vi "LVJSON Load.vi"(8 "error in (no error)":errorcluster, 11 "JSON in":string) -> (0 "error out":errorcluster, 1 "Empty?":bool, 3 "Root Element out":T1)   [LabVIEW 2019, in "labview_json.lvlib"]
uses:
  labview_json.lvlib
  Element.ctl
  Element Type.ctl
  <vilib>/Utility/error.llb/Error Cluster From Error Code.vi
  <vilib>/ErrorRing/Error Ring.xnode
  <vilib>/regexp/Match Regular Expression.xnode
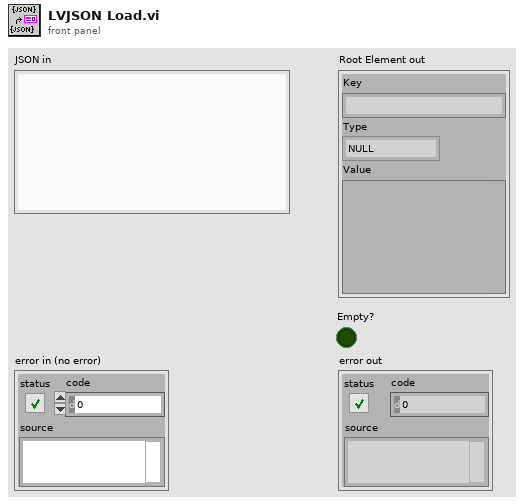
[diagram p1: front panel]
types:
  T1 = typedef "labview_json.lvlib/Element.ctl" = cluster{"Key":string, "Type":T2, "Value":variant}
  T2 = typedef "labview_json.lvlib/Element Type.ctl" = enum8{"NULL", "BOOL", "INT", "UINT", "FLOAT", "STRING", "ARRAY", "OBJECT", "SKIP"}
  T3 = cluster{"Kind":enum8{"Root", "Object", "Array"}, "Name":string, "Values":T1[]}[]
  T4 = cluster{"Kind":enum8{"Root", "Object", "Array"}, "Name":string, "Values":T1[]}
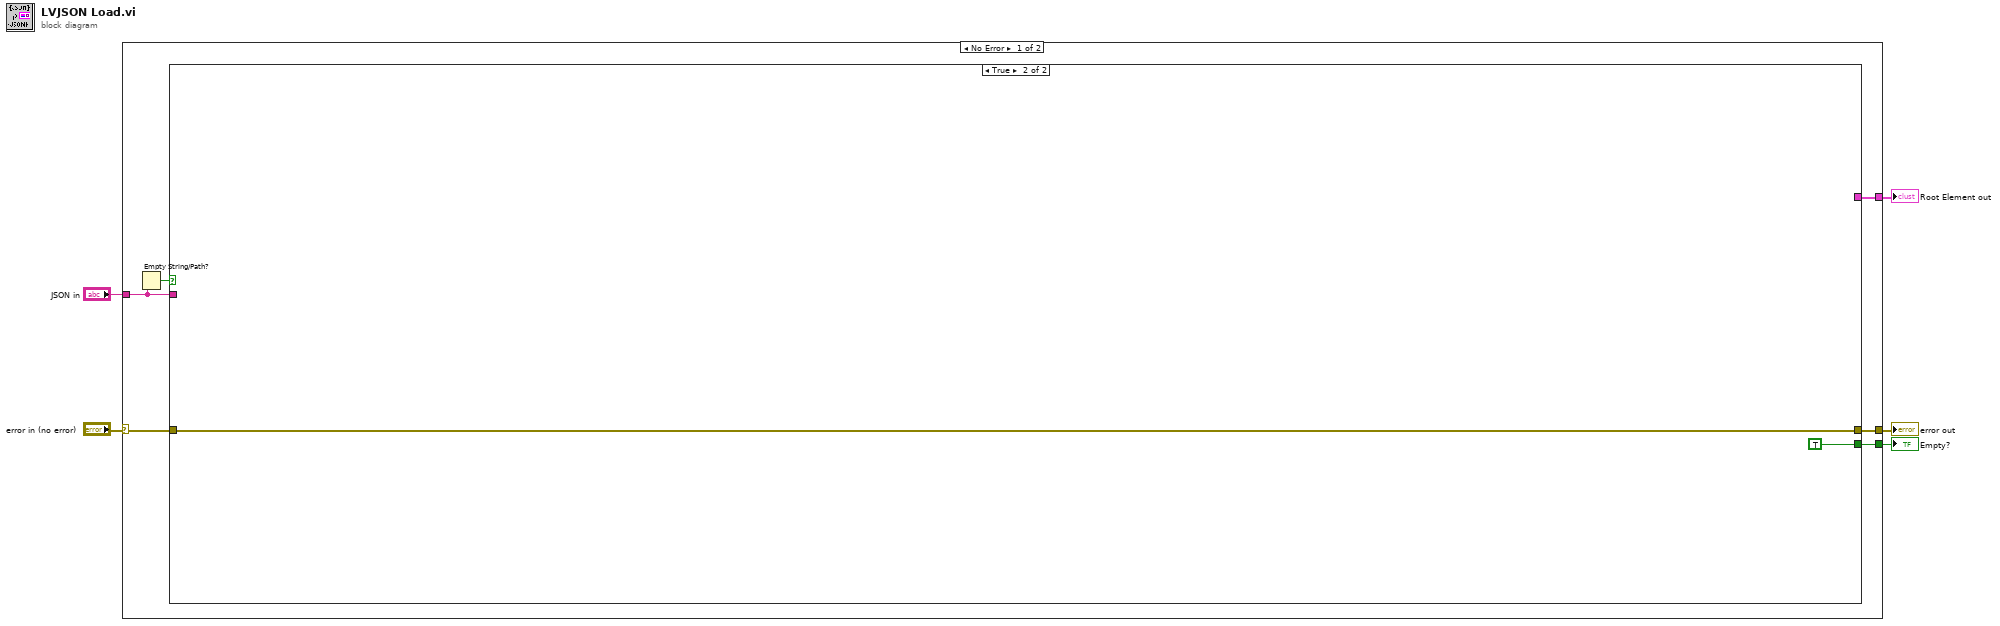
[diagram p0: block diagram]
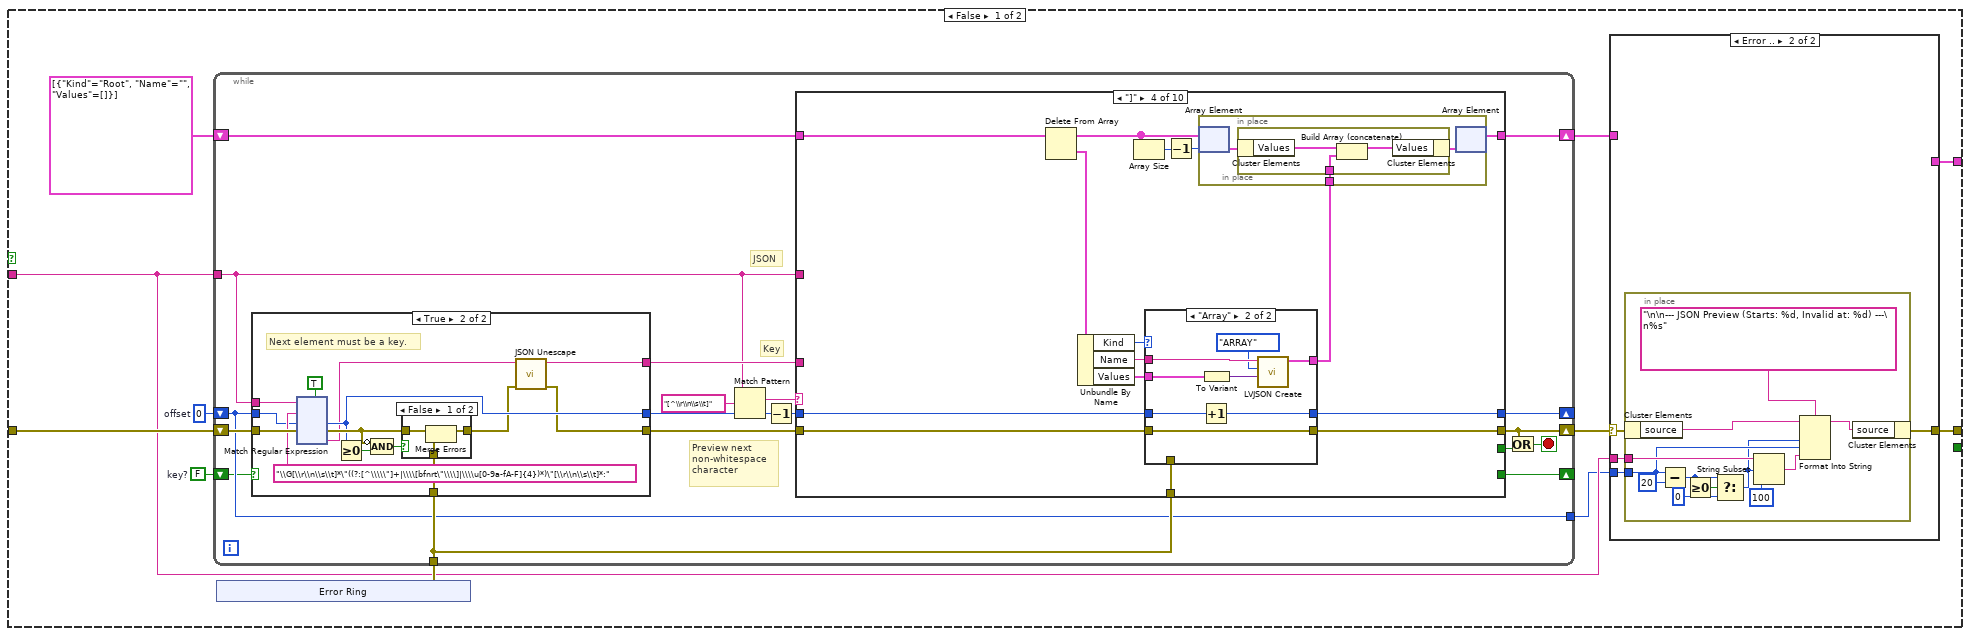
[diagram p2: hidden frame]
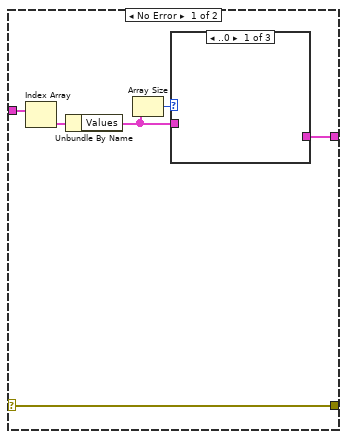
[diagram p3: hidden frame]
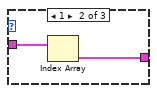
[diagram p4: hidden frame]
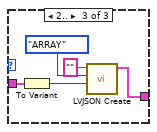
[diagram p5: hidden frame]
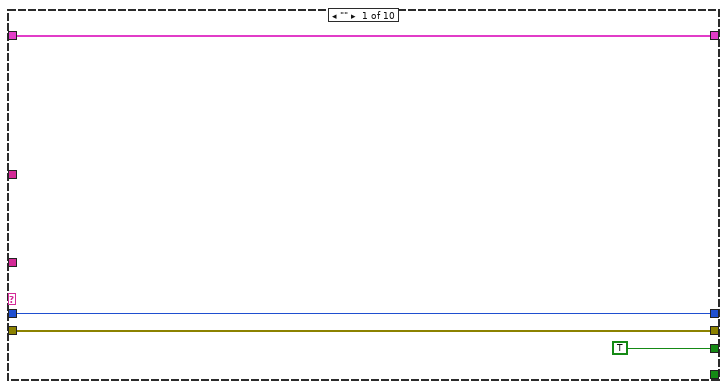
[diagram p8: hidden frame]
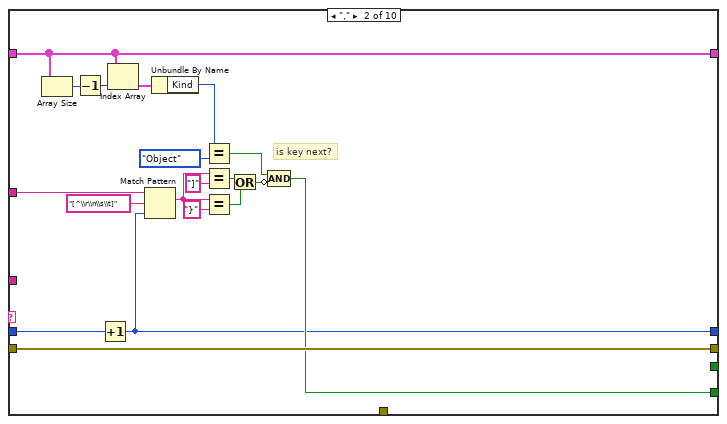
[diagram p9: hidden frame]
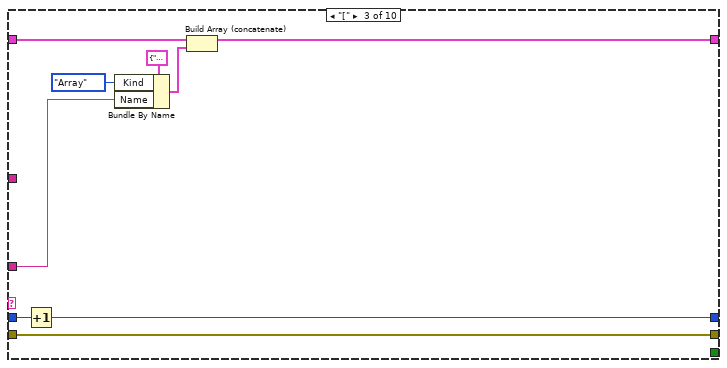
[diagram p10: hidden frame]
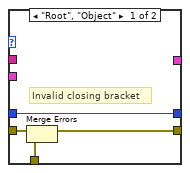
[diagram p11: hidden frame]
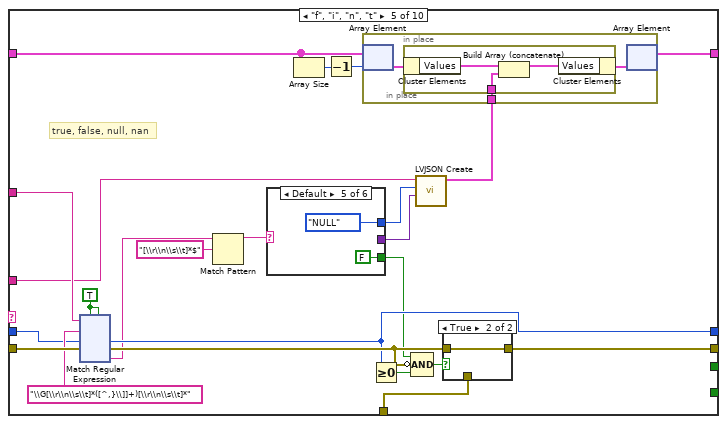
[diagram p12: hidden frame]
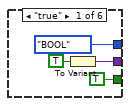
[diagram p13: hidden frame]
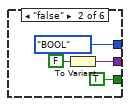
[diagram p14: hidden frame]
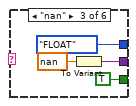
[diagram p15: hidden frame]
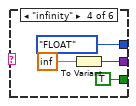
[diagram p16: hidden frame]
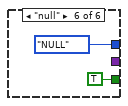
[diagram p17: hidden frame]
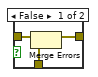
[diagram p18: hidden frame]
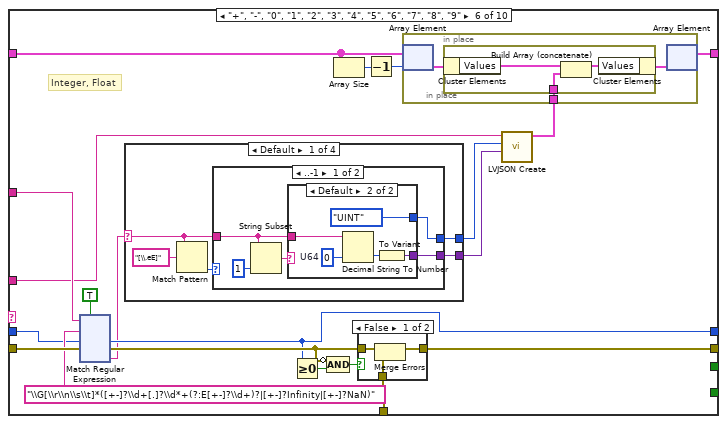
[diagram p19: hidden frame]
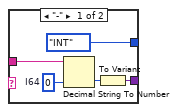
[diagram p20: hidden frame]
diagram:
  n1 = case shown="No Error" "error in (no error)" {
    selector: "error in (no error)" -> [w11 w827]
    tunnel: [w10 _] -> w4
    tunnel: [w9 w827] -> w3
    tunnel: "JSON in" -> [w8 _]
    tunnel: [w6 _] -> w1
    frame No Error {
      n2 = Empty String/Path?(string/path=w8) -> (empty?=w7:bool)
      n3 = case shown="True" w7 {
        tunnel: w11 -> [w21 w826]
        tunnel: [w12 _] -> w10
        tunnel: [w18 w826] -> w9
        tunnel: w8 -> [w16 _]
        tunnel: [_ TRUE] -> w6
        frame False {
          w22 = 0  # offset
          w14 = FALSE  # key?
          n4 = xnode "Error Ring"() -> ("error out"=w20:errorcluster)
          n5 = while {
            tunnel: w16 -> [w64]
            shift-right: [w74] -> w13
            shift-left: T3 [{"Kind"=enum."Root", "Name"="", "Values"=[]}] ("Context") -> [w73]
            shift-right: [w72] -> _
            shift-left: w22 -> [w58]
            shift-right: [w61] -> w17
            shift-left: w21 -> [w71]
            tunnel: w20 -> [w63]
            tunnel: [w58] -> w15
            shift-right: [w56] -> _
            shift-left: w14 -> [w57]
            stop <- w60 stop-if-true
            # "JSON"
            # "Key"
            # "Preview next\nnon-whitespace\ncharacter"
            n6 = case shown="True" w57 {
              tunnel: w64 -> [_ w89]
              tunnel: w71 -> [w76 w88]
              tunnel: w58 -> [w75 w86]
              tunnel: [w76 w77] -> w67
              tunnel: w63 -> [_ w83]
              tunnel: [w75 w81] -> w69
              tunnel: [_ w79] -> w66
              frame False {
                # "No key"
                # "Next element can be anything"
              }
              frame True {
                # "Next element must be a key."
                n7 = xnode "Match Regular Expression"("input string"=w89, "regular expression"="\\G[\\r\\n\\s\\t]*\"((?:[^\\\\\"]+|\\\\[bfnrt\"\\\\]|\\\\u[0-9a-fA-F]{4})*)\"[\\r\\n\\s\\t]*:", "offset (0)"=w86, "error in"=w88, "multiline? (F)"=TRUE) -> ("offset past match"=w81:i32, "error out"=w82:errorcluster, "submatch 1"=w80:string)  [unwired: 1 in, 3 out]
                n8 = Greater Or Equal To 0?(x=w81) -> (x >= 0?=w85:bool)
                n9 = Compound Arithmetic op=AND(invert w82, w85) -> (w84:bool)
                n10 = case shown="False" w84 {
                  tunnel: w83 -> [w91 _]
                  tunnel: w82 -> [w93 w94]
                  tunnel: [w92 w94] -> w78
                  frame False {
                    n11 = Merge Errors(w93, w91) -> (w92:errorcluster)
                  }
                  frame True {
                  }
                }
                n12 = call "JSON Unescape.vi"("error in (no error)"=w78, "Escaped String"=w80) -> ("error out"=w77:errorcluster, "String out"=w79:string)  [unwired: 7 in, 1 out]
              }
            }
            n13 = Match Pattern(string=w64, regular expression="[^\\r\\n\\s\\t]", offset (0)=w69) -> (match substring=w68:string, offset past match=w65:i32)  [unwired: 2 out]
            n14 = Decrement(x=w65) -> (x-1=w62:i32)
            n15 = case shown="\"]\"" w68 {
              tunnel: [TRUE _ _ _ _ _ _ _ _ _] -> w59
              tunnel: w64 -> [_ w219 _ _ w293 w459 w641 w778 _ _]
              tunnel: w62 -> [w212 w218 w237 w245 w284 w450 w634 w781 w789 w822]
              tunnel: [w213 w233 w241 w252 w296 w462 w644 w785 w796 w824] -> w74
              tunnel: w73 -> [w213 w233 w242 w257 w295 w461 w643 w786 w801 w824]
              tunnel: [w212 w215 w235 w246 w286 w452 w636 w774 w790 w822] -> w72
              tunnel: [w211 w217 w236 w249 w285 w451 w635 w780 w793 w821] -> w61
              tunnel: w67 -> [w211 w217 w236 w248 w294 w460 w642 w780 w792 w823]
              tunnel: w66 -> [_ _ w239 _ w279 w448 w629 w783 _ _]
              tunnel: w63 -> [_ _ _ w247 w287 w453 w637 _ w791 w820]
              tunnel: [_ w216 _ _ _ _ _ w775 _ _] -> w56
              frame "" {
              }
              frame "," {
                # "is key next?"
                n16 = Array Size(array=w233) -> (size(s)=w232:i32)
                n17 = Decrement(x=w232) -> (x-1=w231:i32)
                n18 = Increment(x=w218) -> (x+1=w215:i32)
                n19 = Index Array(array=w233, index=w231) -> (element=w230:T4)
                n20 = Match Pattern(string=w219, regular expression="[^\\r\\n\\s\\t]", offset (0)=w215) -> (match substring=w222:string)  [unwired: 3 out]
                n21 = Unbundle By Name(w230) -> ("Kind"=w221:enum8{"Root", "Object", "Array"})
                n22 = Equal?(x=w221, y=enum8{"Root", "Object", "Array"}."Object") -> (x = y?=w225:bool)
                n23 = Equal?(x=w222, y="]") -> (x = y?=w227:bool)
                n24 = Equal?(x=w222, y="}") -> (x = y?=w226:bool)
                n25 = Or(x=w227, y=w226) -> (x .or. y?=w224:bool)
                n26 = Compound Arithmetic op=AND(w225, invert w224) -> (w216:bool)
              }
              frame "[" {
                n27 = Increment(x=w237) -> (x+1=w235:i32)
                n28 = Bundle By Name(cluster=T4 {"Kind"=enum."Root", "Name"="", "Values"=[]} ("Context"), "Kind"=enum8{"Root", "Object", "Array"}."Array", "Name"=w239) -> (w240:T4)
                n29 = Build Array (concatenate)(w242, w240) -> (w241:T3)
              }
              frame "]" {
                n30 = Delete From Array(array=w257) -> (deleted portion=w256:T4, array with subset deleted=w253:T3)  [unwired: 2 in]
                n31 = Unbundle By Name(w256) -> ("Kind"=w251:enum8{"Root", "Object", "Array"}, "Name"=w244:string, "Values"=w250:T1[])
                n32 = Array Size(array=w253) -> (size(s)=w255:i32)
                n33 = case shown="\"Array\"" w251 {
                  tunnel: w250 -> [_ w266]
                  tunnel: [w260 w268] -> w249
                  tunnel: w248 -> [w261 w268]
                  tunnel: w247 -> [w259 _]
                  tunnel: [w258 w267] -> w246
                  tunnel: w245 -> [w258 w269]
                  tunnel: [_ w263] -> w243
                  tunnel: w244 -> [_ w264]
                  frame "Root", "Object" {
                    # "Invalid closing bracket"
                    n34 = Merge Errors(w261, w259) -> (w260:errorcluster)
                  }
                  frame "Array" {
                    n35 = Increment(x=w269) -> (x+1=w267:i32)
                    n36 = To Variant(anything=w266) -> (Variant=w265:variant)
                    n37 = call "LVJSON Create.vi"("Variant (Void=Default Type)"=w265, "Type"=Element_Type."ARRAY", "Key"=w264) -> ("Element out"=w263:T1)  [unwired: 8 in]
                  }
                }
                n38 = Decrement(x=w255) -> (x-1=w254:i32)
                n39 = in-place {
                  in-place-border: w243 -> [w271]
                  n40 = in-place-array #1(w253, w254) -> (w272:T4)
                  n41 = in-place {
                    in-place-border: w271 -> [w273]
                    n42 = in-place-cluster #2(w272) -> ("Values"=w275:T1[])
                    n43 = Build Array (concatenate)(w275, w273) -> (w274:T1[])
                    n44 = in-place-cluster #2("Values"=w274) -> (w270:T4)
                  }
                  n45 = in-place-array #1(w270) -> (w252:T3)  [unwired: 1 out]
                }
              }
              frame "f", "i", "n", "t" {
                w291 = TRUE ("ignore case? (F)")
                # "true, false, null, nan"
                n46 = xnode "Match Regular Expression"("input string"=w293, "regular expression"="\\G[\\r\\n\\s\\t]*([^,}\\]]+)[\\r\\n\\s\\t]*", "offset (0)"=w284, "error in"=w294, "ignore case? (F)"=w291, "multiline? (F)"=w291) -> ("offset past match"=w286:i32, "error out"=w288:errorcluster, "submatch 1"=w281:string)  [unwired: 3 out]
                n47 = Match Pattern(string=w281, regular expression="[\\r\\n\\s\\t]*$") -> (before substring=w280:string)  [unwired: 1 in, 3 out]
                n48 = case shown="Default" w280 {
                  tunnel: [Element_Type."BOOL" ("Type") Element_Type."BOOL" ("Type") Element_Type."FLOAT" ("Type") Element_Type."FLOAT" ("Type") Element_Type."NULL" ("Type") Element_Type."NULL" ("Type")] -> w278
                  tunnel: [w300 w304 w309 w313 _ _] -> w277
                  tunnel: [TRUE TRUE TRUE TRUE FALSE TRUE] -> w283
                  frame "true" {
                    n49 = To Variant(anything=TRUE) -> (Variant=w300:variant)
                  }
                  frame "false" {
                    n50 = To Variant(anything=FALSE) -> (Variant=w304:variant)
                  }
                  frame "nan" {
                    n51 = To Variant(anything=nan) -> (Variant=w309:variant)
                  }
                  frame "infinity" {
                    n52 = To Variant(anything=inf) -> (Variant=w313:variant)
                  }
                  frame Default {
                  }
                  frame "null" {
                  }
                }
                n53 = Array Size(array=w295) -> (size(s)=w298:i32)
                n54 = Decrement(x=w298) -> (x-1=w297:i32)
                n55 = Greater Or Equal To 0?(x=w286) -> (x >= 0?=w289:bool)
                n56 = Compound Arithmetic op=AND(w283, invert w288, w289) -> (w290:bool)
                n57 = call "LVJSON Create.vi"("Variant (Void=Default Type)"=w277, "Type"=w278, "Key"=w279) -> ("Element out"=w276:T1)  [unwired: 8 in]
                n58 = in-place {
                  in-place-border: w276 -> [w440]
                  n59 = in-place-array #3(w295, w297) -> (w441:T4)
                  n60 = in-place {
                    in-place-border: w440 -> [w442]
                    n61 = in-place-cluster #4(w441) -> ("Values"=w444:T1[])
                    n62 = Build Array (concatenate)(w444, w442) -> (w443:T1[])
                    n63 = in-place-cluster #4("Values"=w443) -> (w439:T4)
                  }
                  n64 = in-place-array #3(w439) -> (w296:T3)  [unwired: 1 out]
                }
                n65 = case shown="True" w290 {
                  tunnel: w287 -> [w319 _]
                  tunnel: w288 -> [w321 w322]
                  tunnel: [w320 w322] -> w285
                  frame False {
                    n66 = Merge Errors(w321, w319) -> (w320:errorcluster)
                  }
                  frame True {
                  }
                }
              }
              frame "+", "-", "0", "1", "2", "3", "4", "5", "6", "7", "8", "9" {
                # "Integer, Float"
                n67 = xnode "Match Regular Expression"("input string"=w459, "regular expression"="\\G[\\r\\n\\s\\t]*([+-]?\\d+[.]?\\d*+(?:E[+-]?\\d+)?|[+-]?Infinity|[+-]?NaN)", "offset (0)"=w450, "error in"=w460, "ignore case? (F)"=TRUE) -> ("offset past match"=w452:i32, "error out"=w454:errorcluster, "submatch 1"=w449:string)  [unwired: 1 in, 3 out]
                n68 = case shown="Default" w449 {
                  selector: w449 -> [w467 _ _ _]
                  tunnel: [w465 Element_Type."FLOAT" ("Type") Element_Type."FLOAT" ("Type") Element_Type."FLOAT" ("Type")] -> w447
                  tunnel: [w466 w491 w494 w497] -> w446
                  frame Default {
                    n69 = Match Pattern(string=w467, regular expression="[\\.eE]") -> (offset past match=w469:i32)  [unwired: 1 in, 3 out]
                    n70 = case shown="..-1" w469 {
                      tunnel: w467 -> [w473 w489]
                      tunnel: [w472 w486] -> w466
                      tunnel: [w470 Element_Type."FLOAT" ("Type")] -> w465
                      frame ..-1 {
                        n71 = String Subset(string=w473, length (rest)=1 ("length (rest)")) -> (substring=w471:string)  [unwired: 1 in]
                        n72 = case shown="Default" w471 {
                          tunnel: w473 -> [w479 w484]
                          tunnel: [w476 w481] -> w472
                          tunnel: [Element_Type."INT" ("Type") Element_Type."UINT" ("Type")] -> w470
                          frame "-" {
                            w478 = i64 0  # I64
                            n73 = Decimal String To Number(string=w479, default (0L)=w478) -> (number=w477:i64)  [unwired: 1 in, 1 out]
                            n74 = To Variant(anything=w477) -> (Variant=w476:variant)
                          }
                          frame Default {
                            w483 = u64 0  # U64
                            n75 = Decimal String To Number(string=w484, default (0L)=w483) -> (number=w482:u64)  [unwired: 1 in, 1 out]
                            n76 = To Variant(anything=w482) -> (Variant=w481:variant)
                          }
                        }
                      }
                      frame 0.. {
                        w488 = 0.0  # DBL
                        n77 = Fract/Exp String To Number(string=w489, default (0 dbl)=w488) -> (number=w487:dbl)  [unwired: 2 in, 1 out]
                        n78 = To Variant(anything=w487) -> (Variant=w486:variant)
                      }
                    }
                  }
                  frame "+Infinity", "Infinity" {
                    n79 = To Variant(anything=inf) -> (Variant=w491:variant)
                  }
                  frame "-Infinity" {
                    n80 = To Variant(anything=-inf) -> (Variant=w494:variant)
                  }
                  frame "+NaN", "-NaN", "NaN" {
                    n81 = To Variant(anything=nan) -> (Variant=w497:variant)
                  }
                }
                n82 = Greater Or Equal To 0?(x=w452) -> (x >= 0?=w455:bool)
                n83 = Compound Arithmetic op=AND(invert w454, w455) -> (w456:bool)
                n84 = Array Size(array=w461) -> (size(s)=w464:i32)
                n85 = case shown="False" w456 {
                  tunnel: w453 -> [w499 _]
                  tunnel: w454 -> [w501 w502]
                  tunnel: [w500 w502] -> w451
                  frame False {
                    n86 = Merge Errors(w501, w499) -> (w500:errorcluster)
                  }
                  frame True {
                  }
                }
                n87 = Decrement(x=w464) -> (x-1=w463:i32)
                n88 = call "LVJSON Create.vi"("Variant (Void=Default Type)"=w446, "Type"=w447, "Key"=w448) -> ("Element out"=w445:T1)  [unwired: 8 in]
                n89 = in-place {
                  in-place-border: w445 -> [w620]
                  n90 = in-place-array #5(w461, w463) -> (w621:T4)
                  n91 = in-place {
                    in-place-border: w620 -> [w622]
                    n92 = in-place-cluster #6(w621) -> ("Values"=w624:T1[])
                    n93 = Build Array (concatenate)(w624, w622) -> (w623:T1[])
                    n94 = in-place-cluster #6("Values"=w623) -> (w619:T4)
                  }
                  n95 = in-place-array #5(w619) -> (w462:T3)  [unwired: 1 out]
                }
              }
              frame "\"" {
                # "String"
                n96 = Array Size(array=w643) -> (size(s)=w646:i32)
                n97 = xnode "Match Regular Expression"("input string"=w641, "regular expression"="\\G[\\r\\n\\s\\t]*\"((?:[^\\\\\"]+|\\\\[bfnrt\"\\\\]|\\\\u[0-9a-fA-F]{4})*)\"", "offset (0)"=w634, "error in"=w642, "multiline? (F)"=TRUE ("ignore case? (F)")) -> ("offset past match"=w636:i32, "error out"=w631:errorcluster, "submatch 1"=w632:string)  [unwired: 1 in, 3 out]
                n98 = Decrement(x=w646) -> (x-1=w645:i32)
                n99 = call "JSON Unescape.vi"("error in (no error)"=w631, "Escaped String"=w632) -> ("error out"=w630:errorcluster, "String out"=w627:string)  [unwired: 7 in, 1 out]
                n100 = To Variant(anything=w627) -> (Variant=w625:variant)
                n101 = call "LVJSON Create.vi"("Variant (Void=Default Type)"=w625, "Type"=Element_Type."STRING", "Key"=w629) -> ("Element out"=w626:T1)  [unwired: 8 in]
                n102 = in-place {
                  in-place-border: w626 -> [w768]
                  n103 = in-place-array #7(w643, w645) -> (w769:T4)
                  n104 = in-place {
                    in-place-border: w768 -> [w770]
                    n105 = in-place-cluster #8(w769) -> ("Values"=w772:T1[])
                    n106 = Build Array (concatenate)(w772, w770) -> (w771:T1[])
                    n107 = in-place-cluster #8("Values"=w771) -> (w767:T4)
                  }
                  n108 = in-place-array #7(w767) -> (w644:T3)  [unwired: 1 out]
                }
                n109 = Greater Or Equal To 0?(x=w636) -> (x >= 0?=w638:bool)
                n110 = Compound Arithmetic op=AND(invert w630, w638) -> (w639:bool)
                n111 = case shown="False" w639 {
                  tunnel: w637 -> [w647 _]
                  tunnel: w630 -> [w649 w650]
                  tunnel: [w648 w650] -> w635
                  frame False {
                    n112 = Merge Errors(w649, w647) -> (w648:errorcluster)
                  }
                  frame True {
                  }
                }
              }
              frame "{" {
                # "Is key next?"
                n113 = Increment(x=w781) -> (x+1=w774:i32)
                n114 = Bundle By Name(cluster=T4 {"Kind"=enum."Root", "Name"="", "Values"=[]} ("Context"), "Kind"=enum8{"Root", "Object", "Array"}."Object", "Name"=w783) -> (w784:T4)
                n115 = Match Pattern(string=w778, regular expression="[^\\r\\n\\s\\t]", offset (0)=w774) -> (match substring=w777:string)  [unwired: 3 out]
                n116 = Build Array (concatenate)(w786, w784) -> (w785:T3)
                n117 = Not Equal?(x=w777, y="}") -> (x != y?=w775:bool)
              }
              frame "}" {
                n118 = Delete From Array(array=w801) -> (deleted portion=w800:T4, array with subset deleted=w797:T3)  [unwired: 2 in]
                n119 = Unbundle By Name(w800) -> ("Kind"=w795:enum8{"Root", "Object", "Array"}, "Name"=w788:string, "Values"=w794:T1[])
                n120 = Array Size(array=w797) -> (size(s)=w799:i32)
                n121 = case shown="\"Object\"" w795 {
                  tunnel: w794 -> [_ w810]
                  tunnel: [w804 w812] -> w793
                  tunnel: w792 -> [w805 w812]
                  tunnel: w791 -> [w803 _]
                  tunnel: [w802 w811] -> w790
                  tunnel: w789 -> [w802 w813]
                  tunnel: [_ w806] -> w787
                  tunnel: w788 -> [_ w808]
                  frame "Root", "Array" {
                    # "Invalid closing bracket"
                    n122 = Merge Errors(w805, w803) -> (w804:errorcluster)
                  }
                  frame "Object" {
                    n123 = Increment(x=w813) -> (x+1=w811:i32)
                    n124 = To Variant(anything=w810) -> (Variant=w809:variant)
                    n125 = call "LVJSON Create.vi"("Variant (Void=Default Type)"=w809, "Type"=Element_Type."OBJECT", "Key"=w808) -> ("Element out"=w806:T1)  [unwired: 8 in]
                  }
                }
                n126 = Decrement(x=w799) -> (x-1=w798:i32)
                n127 = in-place {
                  in-place-border: w787 -> [w815]
                  n128 = in-place-array #9(w797, w798) -> (w816:T4)
                  n129 = in-place {
                    in-place-border: w815 -> [w817]
                    n130 = in-place-cluster #10(w816) -> ("Values"=w819:T1[])
                    n131 = Build Array (concatenate)(w819, w817) -> (w818:T1[])
                    n132 = in-place-cluster #10("Values"=w818) -> (w814:T4)
                  }
                  n133 = in-place-array #9(w814) -> (w796:T3)  [unwired: 1 out]
                }
              }
              frame Default {
                # "Invalid value"
                n134 = Merge Errors(w823, w820) -> (w821:errorcluster)
              }
            }
            n135 = Or(x=w61, y=w59) -> (x .or. y?=w60:bool)
          }
          n136 = case shown="Error .." w17 {
            selector: w17 -> [w28 w39]
            tunnel: [w28 w36] -> w18
            tunnel: w16 -> [_ w38]
            tunnel: w15 -> [_ w37]
            tunnel: w13 -> [w24 _]
            tunnel: [w23 _] -> w12
            frame No Error {
              n137 = Index Array(array=w24) -> (element=w26:T4)  [unwired: 1 in]
              n138 = Unbundle By Name(w26) -> ("Values"=w25:T1[])
              n139 = Array Size(array=w25) -> (size(s)=w27:i32)
              n140 = case shown="..0" w27 {
                tunnel: w25 -> [_ w30 w35]
                tunnel: [_ w29 w31] -> w23
                frame ..0 {
                }
                frame 1 {
                  n141 = Index Array(array=w30) -> (element=w29:T1)  [unwired: 1 in]
                }
                frame 2.. {
                  n142 = To Variant(anything=w35) -> (Variant=w34:variant)
                  n143 = call "LVJSON Create.vi"("Variant (Void=Default Type)"=w34, "Type"=Element_Type."ARRAY", "Key"="") -> ("Element out"=w31:T1)  [unwired: 8 in]
                }
              }
            }
            frame Error {
              n144 = in-place {
                in-place-border: w38 -> [w51]
                in-place-border: w37 -> [w41]
                n145 = in-place-cluster #11(w39) -> ("source"=w48:string)
                n146 = Subtract(x=w41, y=20 ("x")) -> (x-y=w44:i32)
                n147 = Greater Or Equal To 0?(x=w44) -> (x >= 0?=w45:bool)
                n148 = Select(t=w44, s=w45, f=0) -> (s? t:f=w40:i32)
                n149 = String Subset(string=w51, offset (0)=w40, length (rest)=100 ("length (rest)")) -> (substring=w42:string)
                n150 = Format Into String(format string="\n\n--- JSON Preview (Starts: %d, Invalid at: %d) ---\n%s", initial string=w48, w40, w41, w42) -> (resulting string=w47:string)  [unwired: 1 in, 1 out]
                n151 = in-place-cluster #11("source"=w47) -> (w36:errorcluster)
              }
            }
          }
        }
        frame True {
        }
      }
    }
    frame Error {
    }
  }
  "Root Element out" <- w4
  "error out" <- w3
  "Empty?" <- w1
